vi "Scan Engine Change Module.vi"(7 "SubPanel Event":refnum<user-event>, 8 "error in (no error)":errorcluster, 9 "SubPanel Ref":refnum<vi>, 10 "Module Model":T1, 11 "Node Ptr In":T2 format="%.0x") -> (0 "error out":errorcluster, 3 "Node Ptr Out":T2 format="%.0x")   [LabVIEW 2011, in "Scan Engine Custom Device.lvlib"]
uses:
  Scan Engine Custom Device.lvlib
  <vilib>/NI Veristand/Custom Device API/Custom Device Item Ref.ctl
  Modules.lvlibp/RSI Module/Module Models.ctl
  Modules.lvlibp/RSI Module/SubPanel Command.ctl
  Modules.lvlibp/RSI Module/RSI Module.lvclass
  <vilib>/NI Veristand/Custom Device API/Custom Device API.lvlib
  Modules.lvlibp
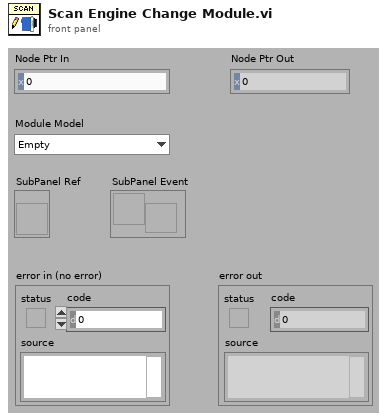
[diagram p1: front panel]
types:
  T1 = typedef "Modules.lvlibp/RSI Module.lvclass/Module Models.ctl" = enum16{"Empty", "NI 9201", "NI 9203", "NI 9205", "NI 9206", "NI 9207", "NI 9208", "NI 9211", "NI 9213", "NI 9214", "NI 9215", "NI 9217", "NI 9219", "NI 9221", "NI 9225", "NI 9227", "NI 9229", "NI 9233", "NI 9234", "NI 9235", "NI 9236", "NI 9237", "NI 9239", "NI 9263", "NI 9264", "NI 9265", "NI 9269", "NI 9375", "NI 9401", "NI 9402", "NI 9403", "NI 9411", "NI 9421", "NI 9422", "NI 9423", "NI 9425", "NI 9426", "NI 9435", "NI 9472", "NI 9474", "NI 9475", "NI 9476", "NI 9477", "NI 9478", "NI 9481", "NI 9482", "NI 9485"}
  T2 = typedef "Custom Device API.lvlib/Custom Device Item Ref.ctl" = u64
  T3 = typedef "Modules.lvlibp/RSI Module.lvclass/SubPanel Command.ctl" = enum16{"Stop"}
  T4 = typedef "Modules.lvlibp/Custom Device API.lvlib/Custom Device Item Ref.ctl" = u64
  T5 = typedef "Modules.lvlibp/RSI Module.lvclass/Slot Settings.ctl" = cluster{"Slot":u32, "EtherCAT?":bool}
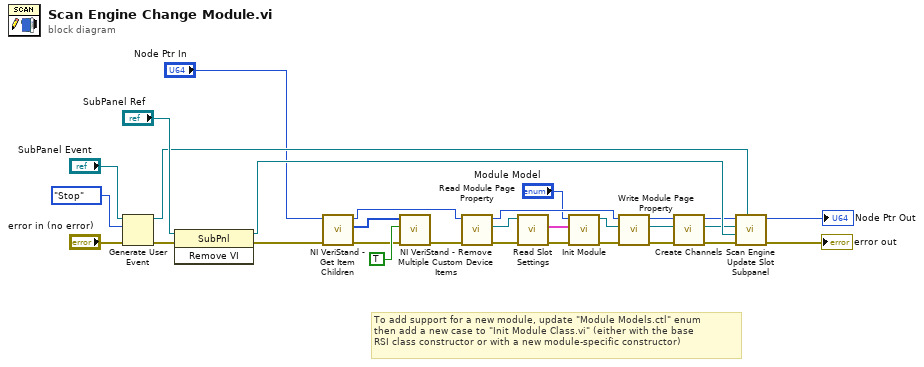
[diagram p0: block diagram]
diagram:
  # "To add support for a new module, update \"Module Models.ctl\" enum\nthen add a new case to \"Init Module Class.vi\" (either with the base\nRSI class constructor or with a new module-specific constructor)"
  n1 = Generate User Event(user event="SubPanel Event", event data cluster=SubPanel_Command."Stop" ("event data"), error in="error in (no error)") -> (user event out=w27:refnum<user-event>, error out=w24:errorcluster)
  n2 = invoke class="SubPnl" method="Remove VI"(reference="SubPanel Ref", error in=w24) -> (reference out=w28:refnum<vi>, error out=w14:errorcluster)  [unwired: 1 in, 1 out]
  n3 = call <vilib>:"NI VeriStand - Get Item Children.vi"("error in (no error)"=w14, "Item Ref in"="Node Ptr In") -> ("error out"=w11:errorcluster, "Child Refs"=w13:T2[], "Item Ref out"=w10:T2)  [unwired: 6 in, 1 out]
  n4 = call <vilib>:"NI VeriStand - Remove Multiple Custom Device Items.vi"("error in (no error)"=w11, "Force Delete (F)"=TRUE, "Item Refs in"=w13) -> ("error out"=w9:errorcluster)  [unwired: 7 in, 1 out]
  n5 = call "Read Module Page Property.vi"("error in (no error)"=w9, "Node Ptr In"=w10) -> ("error out"=w23:errorcluster, "RSI Module"=w22:refnum<class "RSI Module.lvclass">, "Node Ptr Out"=w21:T4)  [unwired: 7 in]
  n6 = call "Read Slot Settings.vi"("error in (no error)"=w23, "RSI Module in"=w22) -> ("error out"=w20:errorcluster, "Slot Settings"=w18:T5)  [unwired: 7 in, 1 out]
  n7 = call "Init Module.vi"("error in (no error)"=w20, "Slot Settings"=w18, "Module Model"="Module Model") -> ("error out"=w16:errorcluster, "RSI Module out"=w17:refnum<class "RSI Module.lvclass">)  [unwired: 7 in]
  n8 = call "Write Module Page Property.vi"("error in (no error)"=w16, "RSI Module"=w17, "Node Ptr In"=w21) -> ("error out"=w8:errorcluster, "RSI Module out"=w6:refnum<class "RSI Module.lvclass">, "Node Ptr Out"=w5:T4)  [unwired: 6 in]
  n9 = call-dynamic "Create Channels.vi"("error in (no error)"=w8, "RSI Module in"=w6, "Parent Ref in"=w5) -> ("error out"=w7:errorcluster, "RSI Module out"=w4:refnum<class "RSI Module.lvclass">, "Parent Ref out"=w3:T4)  [unwired: 6 in]
  n10 = call "Scan Engine Update Slot Subpanel.vi"("SubPanel Event"=w27, "error in (no error)"=w7, "SubPanel Ref"=w28, "RSI Module in"=w4, "Node Ptr In"=w3) -> ("error out"=→"error out":errorcluster, "Node Ptr Out"=→"Node Ptr Out":T2)  [unwired: 4 in, 1 out]
